vi "MotorWait2.vi"(8 "error in (no error)":errorcluster, 9 "Intended Position":dbl[](array[numeric]), 10 "N Ax":dbl, 11 "CU ID":i32) -> (0 "error out":errorcluster)   [LabVIEW 2021]
panel:
  out "Error":dbl
  in  "Tolerance":dbl=0.0006
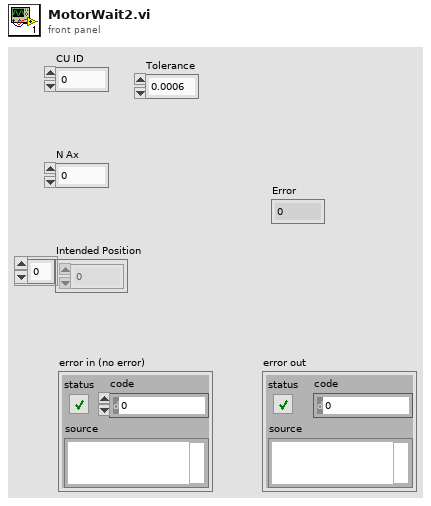
[diagram p1: front panel]
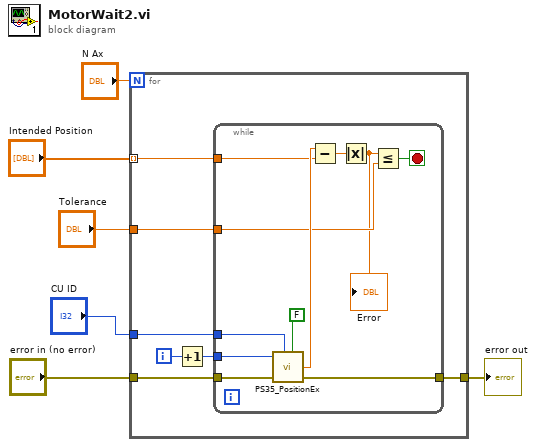
[diagram p0: block diagram]
diagram:
  n1 = for {
    N: "N Ax" -> [_]
    tunnel: "CU ID" -> [w11]
    tunnel: "error in (no error)" -> [w10]
    tunnel: [w9] -> w6
    tunnel: "Intended Position" -> [w8] mode=indexing
    tunnel: "Tolerance" -> [w7]
    i -> [w13]
    n2 = Increment(x=w13) -> (x+1=w12:i32)
    n3 = while {
      tunnel: w12 -> [w23]
      tunnel: w11 -> [w24]
      tunnel: w10 -> [w21]
      tunnel: [w19] -> w9
      tunnel: w8 -> [w18]
      tunnel: w7 -> [w16]
      stop <- w17 stop-if-true
      n4 = call "PS35_PositionEx.vi"("Axis number"=w23, "Control unit ID"=w24, "error in (no error)"=w21, "function"=FALSE) -> ("dValue-Out"=w20:dbl, "error out"=w19:errorcluster)  [unwired: 4 in]
      n5 = Subtract(x=w20, y=w18) -> (x-y=w15:dbl)
      n6 = Absolute Value(x=w15) -> (abs(x)=w14:dbl)
      "Error" <- w14
      n7 = Less Or Equal?(x=w14, y=w16) -> (x <= y?=w17:bool)
    }
  }
  "error out" <- w6
